vi "Ring (SubVI).vi"(8 "error in":errorcluster, 10 "Ref":T1, 11 "paramUnicorn":T2={"conParam"={"ReadIntParam"=FALSE, "ReadDescrParam"=FALSE, "ReadFloatParam"=FALSE, "debug"=FALSE, "ReadJSON"=FALSE, "IP_address"="", "N_attempts"=0, "type_con"=enum."Serial", "MB_address"=0, "VISA"="", "connection ID"=refnum, "nameDevices"="", "timeout"=0, "port"=0, "type_version"="", "baud_rate"=0, "VersionControl"=FALSE, "TCP_conn"=FALSE, "WindowSize"=700}, "Param"={"NumParam"={"NTelem"=0, "NInt"=0, "NFloat"=0, "NTable"=0}, "ParamInt"=[], "Telemetry"=[], "Table"=[], "ParamFloat"=[]}}) -> (0 "error out":errorcluster)   [LabVIEW 2017, in "LV_Unicorn.lvlib"]
uses:
  LV_Unicorn.lvlib
  Control/unicorn_Param.ctl
  Control/unicorn_conn.ctl
  Control/unicorn_JSON.ctl
  Control/unicorn_ParamInt.ctl
  Control/unicorn_Telemetry.ctl
  Control/unicorn_Table.ctl
  Control/unicorn_ParamFloat.ctl
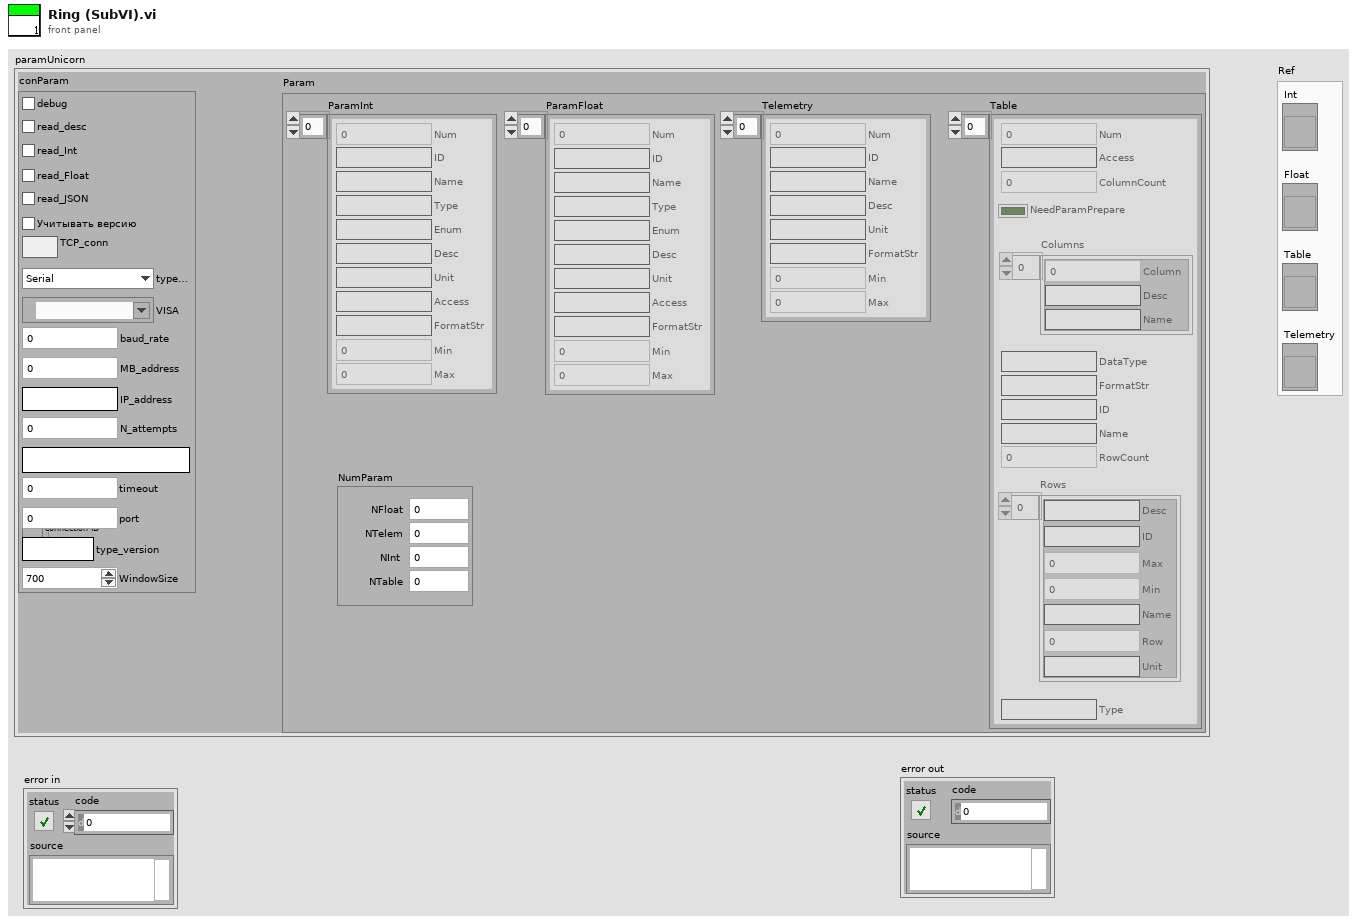
[diagram p1: front panel]
types:
  T1 = cluster{"Int":refnum<vi>, "Float":refnum<vi>, "Table":refnum<vi>, "Telemetry":refnum<vi>}
  T2 = typedef "LV_Unicorn.lvlib/unicorn_Param.ctl" = cluster{"conParam":T3, "Param":T4}
  T3 = typedef "LV_Unicorn.lvlib/unicorn_conn.ctl" = cluster{"ReadIntParam":bool, "ReadDescrParam":bool, "ReadFloatParam":bool, "debug":bool, "ReadJSON":bool, "IP_address":string, "N_attempts":i32, "type_con":enum16{"Serial", "TCP"}, "MB_address":i32, "VISA":refnum<visa-resource-name>, "connection ID":refnum<k5>, "nameDevices":string, "timeout":i32, "port":u16, "type_version":string, "baud_rate":u32, "VersionControl":bool, "TCP_conn":bool, "WindowSize":i32}
  T4 = typedef "LV_Unicorn.lvlib/unicorn_JSON.ctl" = cluster{"NumParam":cluster{"NTelem":i32, "NInt":i32, "NFloat":i32, "NTable":i32}, "ParamInt":T5, "Telemetry":T6, "Table":T7, "ParamFloat":T8}
  T5 = typedef "LV_Unicorn.lvlib/unicorn_ParamInt.ctl" = cluster{"ID":string, "Num":i32, "Name":string, "Type":string, "Enum":string, "Desc":string, "Unit":string, "Access":string, "FormatStr":string, "Min":i32, "Max":i32}[]
  T6 = typedef "LV_Unicorn.lvlib/unicorn_Telemetry.ctl" = cluster{"ID":string, "Num":i32, "Name":string, "Desc":string, "Unit":string, "FormatStr":string, "Min":i32, "Max":i32}[]
  T7 = typedef "LV_Unicorn.lvlib/unicorn_Table.ctl" = cluster{"Num":i32, "Access":string, "ColumnCount":i32, "NeedParamPrepare":bool, "Columns":cluster{"Column":i32, "Desc":string, "Name":string}[], "DataType":string, "FormatStr":string, "ID":string, "Name":string, "RowCount":i32, "Rows":cluster{"Desc":string, "ID":string, "Max":i32, "Min":i32, "Name":string, "Row":i32, "Unit":string}[], "Type":string}[]
  T8 = typedef "LV_Unicorn.lvlib/unicorn_ParamFloat.ctl" = cluster{"ID":string, "Num":i32, "Name":string, "Type":string, "Enum":string, "Desc":string, "Unit":string, "Access":string, "FormatStr":string, "Min":sgl, "Max":sgl}[]
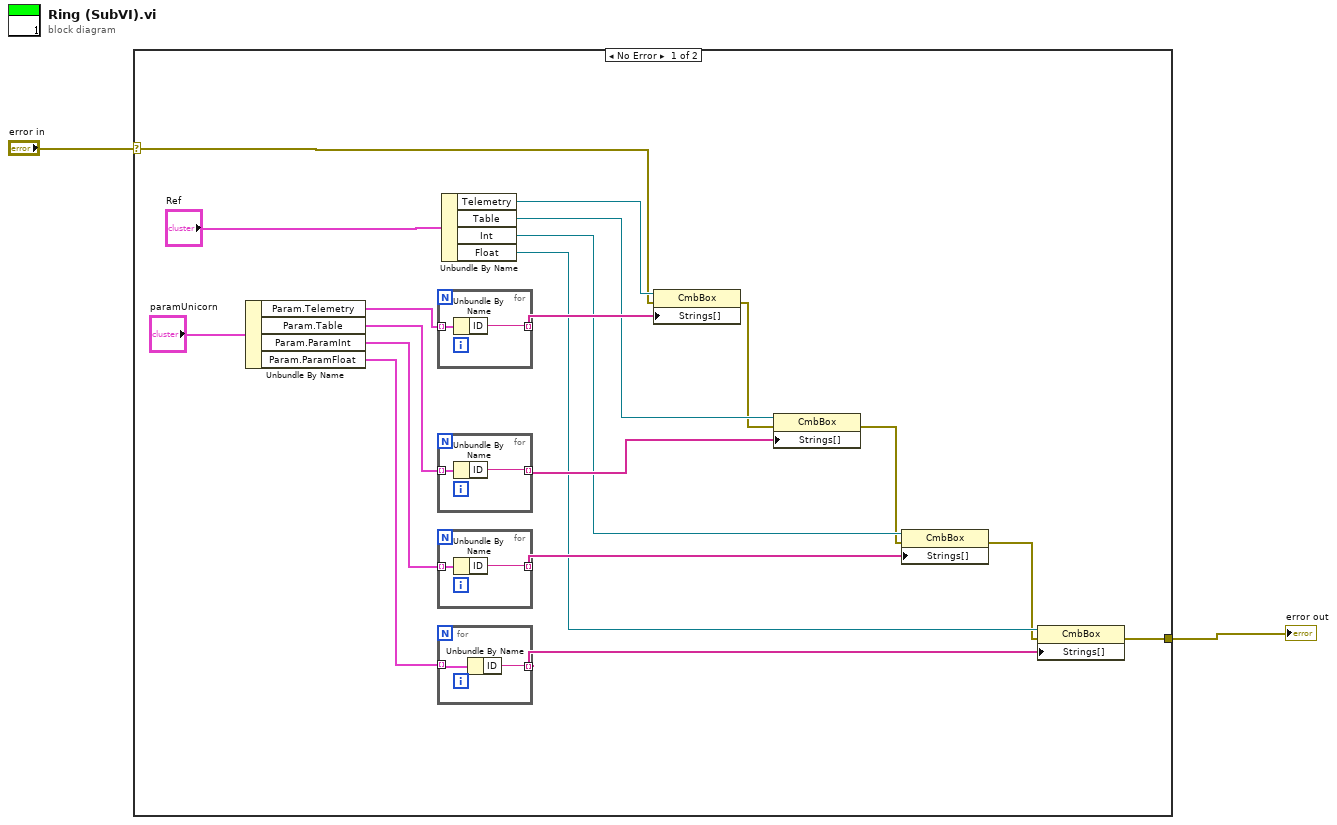
[diagram p0: block diagram]
diagram:
  n1 = case shown="No Error" "error in" {
    selector: "error in" -> [w3 w30]
    tunnel: [w4 w30] -> w2
    frame No Error {
      n2 = Unbundle By Name("paramUnicorn") -> ("Param.Telemetry"=w20:T6, "Param.Table"=w18:T7, "Param.ParamInt"=w16:T5, "Param.ParamFloat"=w14:T8)
      n3 = for {
        tunnel: w20 -> [w23] mode=indexing
        tunnel: [w22] -> w21 mode=indexing
        n4 = Unbundle By Name(w23) -> ("ID"=w22:string)
      }
      n5 = for {
        tunnel: w18 -> [w25] mode=indexing
        tunnel: [w24] -> w19 mode=indexing
        n6 = Unbundle By Name(w25) -> ("ID"=w24:string)
      }
      n7 = for {
        tunnel: w16 -> [w27] mode=indexing
        tunnel: [w26] -> w17 mode=indexing
        n8 = Unbundle By Name(w27) -> ("ID"=w26:string)
      }
      n9 = for {
        tunnel: w14 -> [w29] mode=indexing
        tunnel: [w28] -> w15 mode=indexing
        n10 = Unbundle By Name(w29) -> ("ID"=w28:string)
      }
      n11 = Unbundle By Name("Ref") -> ("Telemetry"=w11:refnum<vi>, "Table"=w10:refnum<vi>, "Int"=w9:refnum<vi>, "Float"=w8:refnum<vi>)
      n12 = property on="Property Node" class="CmbBox"(reference=w11, error in=w3, "Strings[]"=w21) -> (error out=w7:errorcluster)  [unwired: 1 out]
      n13 = property on="Property Node" class="CmbBox"(reference=w10, error in=w7, "Strings[]"=w19) -> (error out=w6:errorcluster)  [unwired: 1 out]
      n14 = property on="Property Node" class="CmbBox"(reference=w9, error in=w6, "Strings[]"=w17) -> (error out=w5:errorcluster)  [unwired: 1 out]
      n15 = property on="Property Node" class="CmbBox"(reference=w8, error in=w5, "Strings[]"=w15) -> (error out=w4:errorcluster)  [unwired: 1 out]
    }
    frame Error {
    }
  }
  "error out" <- w2
